vi "Populate Ctrl.vi"(8 "error in (no error)":errorcluster, 11 "Composed Field in":refnum<class "Composed Field.lvclass">) -> (0 "error out":errorcluster, 3 "Composed Field out":refnum<class "Composed Field.lvclass">)   [LabVIEW 2020]
uses:
  Column/Composed Column.lvclass
  Ring Ctrl Value Source/Ring Ctrl Value Source.lvclass
  Composed Field.lvclass
  C:/Users/User/Desktop/Raman Program/Database OOP/source/Database OOP/Column Libraries/Column/Composed Column.lvclass
  C:/Users/User/Desktop/Raman Program/Database OOP/source/Database OOP/Column Libraries/Column Interface/Column Interface Class/Column Interface.lvclass
  C:/Users/User/Desktop/Raman Program/Database OOP/source/Database OOP/Column Libraries/Field Interfaces/Field Interface Class/Field Interface.lvclass
  C:/Users/User/Desktop/Raman Program/Database OOP/source/Database OOP/Column Libraries/Composed Field/Composed Field.lvclass
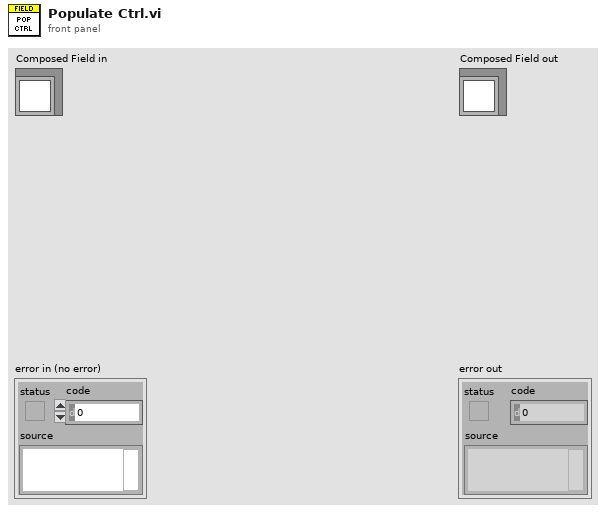
[diagram p1: front panel]
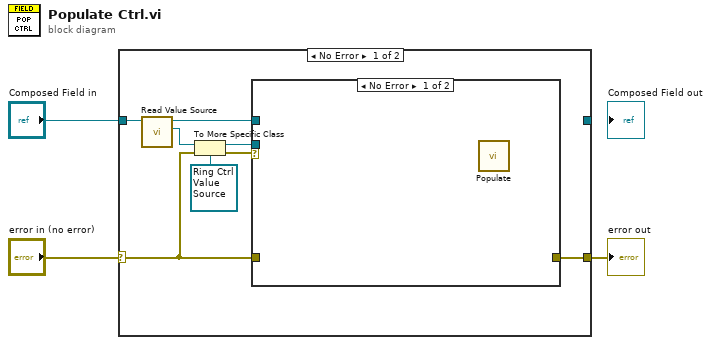
[diagram p0: block diagram]
diagram:
  n1 = case shown="No Error" "error in (no error)" {
    selector: "error in (no error)" -> [w7 w14]
    tunnel: [w6 w14] -> w2
    tunnel: "Composed Field in" -> [w11 w13]
    tunnel: [_ w13] -> _
    frame No Error {
      n2 = call "Read Value Source.vi"("Composed Column in"=w11) -> ("Value Source"=w10:refnum<class "Value Source.lvclass">, "Composed Column out"=w5:refnum<class "Composed Field.lvclass">)  [unwired: 8 in, 1 out]
      n3 = To More Specific Class(target class=refnum<class "Ring Ctrl Value Source.lvclass"> refnum ("Composed Columns.lvlib:Ring Ctrl Value Source.lvclass"), reference=w10, error in=w7) -> (specific class reference=w4:refnum<class "Ring Ctrl Value Source.lvclass">, error out=w8:errorcluster)
      n4 = case shown="No Error" w8 {
        tunnel: w7 -> [_ w12]
        tunnel: [_ w12] -> w6
        tunnel: w5 -> [_ _]
        tunnel: w4 -> [_ _]
        frame No Error {
          n5 = call-dynamic "Populate.vi"() -> ()  [unwired: 10 in, 2 out]
        }
        frame Error {
        }
      }
    }
    frame Error {
    }
  }
  "error out" <- w2
